vi "Transceiver Thread.New.vi"(8 "error in (no error)":errorcluster, 9 "Debug Flags":refnum<class "Debug Flags.lvclass">, 10 "Transfer Groups":refnum<class "Transfer Group.lvclass">[](array[class]), 11 "Transceiver type":refnum<class "Transceiver.lvclass">) -> (0 "error out":errorcluster, 3 "Transceiver Thread out":refnum<class "Transceiver Thread.lvclass">)   [LabVIEW 2017, in "DSF.Engine.lvlib" / "Transceiver Thread.lvclass"]
uses:
  Transceiver Thread.lvclass
  Transceiver.lvclass
  Debug/Debug Flags.lvclass
  Transfer/Transfer Group.lvclass
  Transceiver Thread.lvclass/Transceiver Thread.ctl
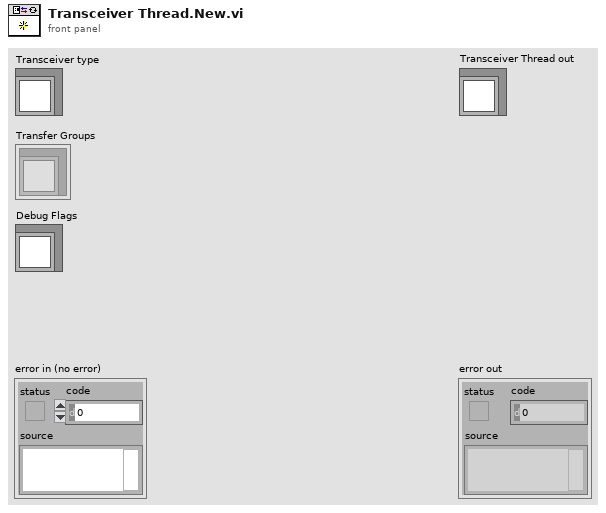
[diagram p1: front panel]
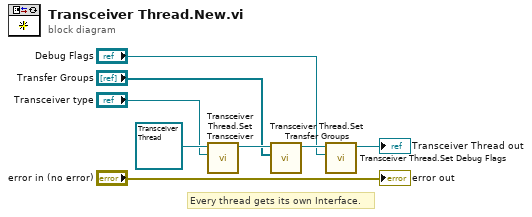
[diagram p0: block diagram]
diagram:
  # "Every thread gets its own Interface."
  n1 = call "Transceiver Thread.Set Transceiver.vi"("Transceiver"="Transceiver type", "Transceiver Thread in"=refnum<class "Transceiver Thread.lvclass"> refnum) -> ("Transceiver Thread out"=w2:refnum<class "Transceiver Thread.lvclass">)  [unwired: 9 in]
  n2 = call "Transceiver Thread.Set Transfer Groups.vi"("Transfer Groups"="Transfer Groups", "Transceiver Thread in"=w2) -> ("Transceiver Thread out"=w6:refnum<class "Transceiver Thread.lvclass">)  [unwired: 9 in]
  n3 = call "Transceiver Thread.Set Debug Flags.vi"("Debug Flags"="Debug Flags", "Transceiver Thread in"=w6) -> ("Transceiver Thread out"=→"Transceiver Thread out":refnum<class "Transceiver Thread.lvclass">)  [unwired: 9 in]
  "error out" <- "error in (no error)"
